vi "spec_set_deflection.vi"(8 "error in (no error)":errorcluster, 9 "deflection value":u32, 10 "detector name":string, 11 "Qtegra in":refnum<class "Qtegra.lvclass">) -> (0 "error out":errorcluster, 2 "return value":string, 3 "Qtegra out":refnum<class "Qtegra.lvclass">)   [LabVIEW 2017, in "Qtegra.lvclass"]
doc: "set the deflection voltage of the detector"
uses:
  Qtegra.lvclass
  \\Mac\Home/my data/University/Lamont/Software/LabView/MSControlSuite_Code/MSControl/Classes/Instrument/instrument.lvclass
  global variables.vi
  instrument.lvclass
  StatusLog/StatusLog.lvclass
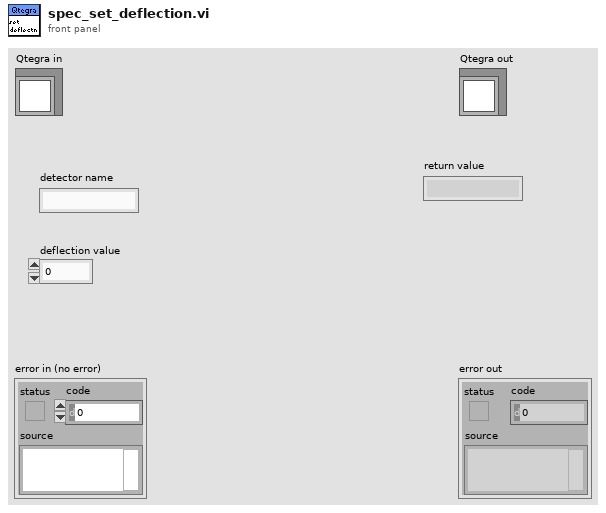
[diagram p1: front panel]
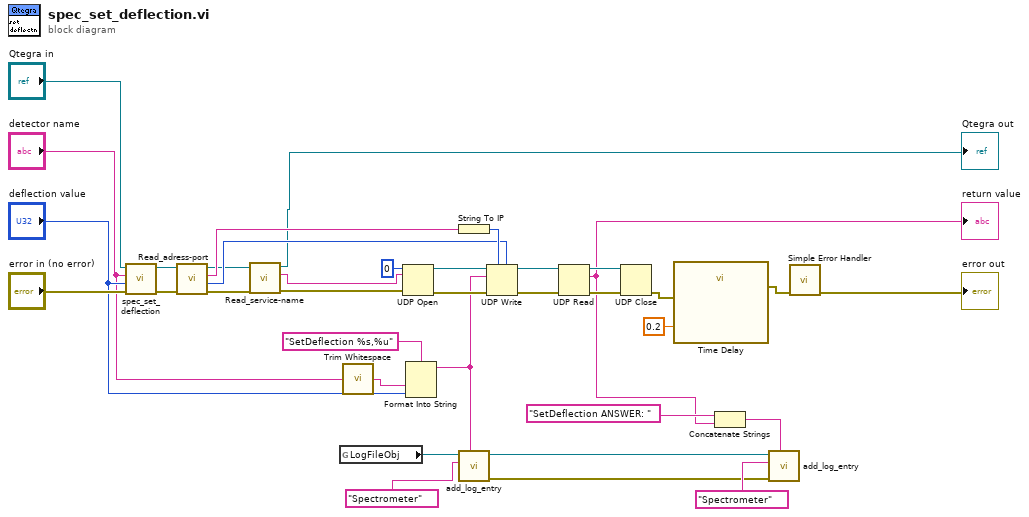
[diagram p0: block diagram]
diagram:
  n1 = call-parent "spec_set_deflection.vi"("error in (no error)"="error in (no error)", "deflection value"="deflection value", "detector name"="detector name", "instrument in"="Qtegra in") -> ("error out"=w7:errorcluster, "instrument out"=w8:refnum<class "Qtegra.lvclass">)  [unwired: 5 in, 1 out]
  n2 = call "Read_adress-port.vi"("error in (no error)"=w7, "instrument in"=w8) -> ("error out"=w26:errorcluster, "port number"=w27:i32, "adress"=w34:string, "instrument out"=w25:refnum<class "Qtegra.lvclass">)  [unwired: 6 in]
  n3 = call-dynamic "Read_service-name.vi"("error in (no error)"=w26, "instrument in"=w25) -> ("error out"=w24:errorcluster, "service name"=w23:string, "instrument out"=→"Qtegra out":refnum<class "Qtegra.lvclass">)  [unwired: 7 in]
  n4 = global read "global variables.vi" "LogFileObj"() -> (w13:refnum<class "StatusLog.lvclass">)
  n5 = call <vilib>:"Trim Whitespace.vi"("string"="detector name") -> ("trimmed string"=w2:string)  [unwired: 1 in]
  n6 = UDP Open(8:w24, 10:w23, 11:u16 0 ("port")) -> (port=w30:refnum<k16>, 0:w31:errorcluster)  [unwired: 2 in, 1 out]
  n7 = Format Into String(format string="SetDeflection %s,%u", w2, "deflection value") -> (resulting string=w15:string)  [unwired: 2 in, 1 out]
  n8 = String To IP(1:w34) -> (0:w33:u32)
  n9 = call-dynamic "add_log_entry.vi"("new entry"=w15, "log identifiers"="Spectrometer", "StatusLog in"=w13) -> ("error out"=w9:errorcluster, "StatusLog out"=w12:refnum<class "StatusLog.lvclass">)  [unwired: 5 in]
  n10 = UDP Write(address=w33, port or service name=w27, connection ID=w30, data in=w15, 8:w31) -> (error out=w28:errorcluster, 3:w29:refnum<k16>)  [unwired: 1 in]
  n11 = UDP Read(connection ID=w29, 8:w28) -> (data out=w5:string, error out=w21:errorcluster, 3:w20:refnum<k16>)  [unwired: 2 in, 2 out]
  "return value" <- w5
  n12 = UDP Close(connection ID=w20, 8:w21) -> (error out=w19:errorcluster)  [unwired: 1 out]
  n13 = call "Time Delay"("error in (no error)"=w19, "Delay Time (s)"=0.2) -> ("error out"=w18:errorcluster)  [unwired: 9 in]
  n14 = Concatenate Strings("SetDeflection ANSWER: ", w5) -> (w10:string)
  n15 = call-dynamic "add_log_entry.vi"("new entry"=w10, "error in (no error)"=w9, "log identifiers"="Spectrometer", "StatusLog in"=w12) -> ()  [unwired: 4 in, 2 out]
  n16 = call <vilib>:"Simple Error Handler.vi"("error in (no error)"=w18) -> ("error out"=→"error out":errorcluster)  [unwired: 4 in, 4 out]
